vi "Get Category.vi"(8 "error in (no error)":errorcluster, 11 "FPGA Module editor node in":refnum<class "FPGA Module editor node.lvclass">) -> (0 "error out":errorcluster, 2 "Category":string, 3 "FPGA Module editor node out":refnum<class "FPGA Module editor node.lvclass">)   [LabVIEW 2014, in "FPGA Module editor node.lvclass"]
uses:
  FPGA Module editor node.lvclass
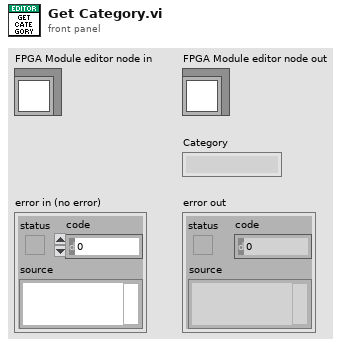
[diagram p1: front panel]
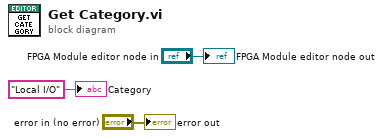
[diagram p0: block diagram]
diagram:
  "error out" <- "error in (no error)"
  "FPGA Module editor node out" <- "FPGA Module editor node in"
  "Category" <- "Local I/O" ("Category")
